vi "Save Report.vi"(8 "error in (no error)":errorcluster, 10 "Results File Location:":path, 11 "NI_report in":refnum<class "NI_report.lvclass">) -> (0 "error out":errorcluster, 1 "generated path":path, 2 "appended path":path, 3 "NI_report out":refnum<class "NI_report.lvclass">)   [LabVIEW 2018]
uses:
  <vilib>/Utility/NIReport.llb/NI_report.lvclass
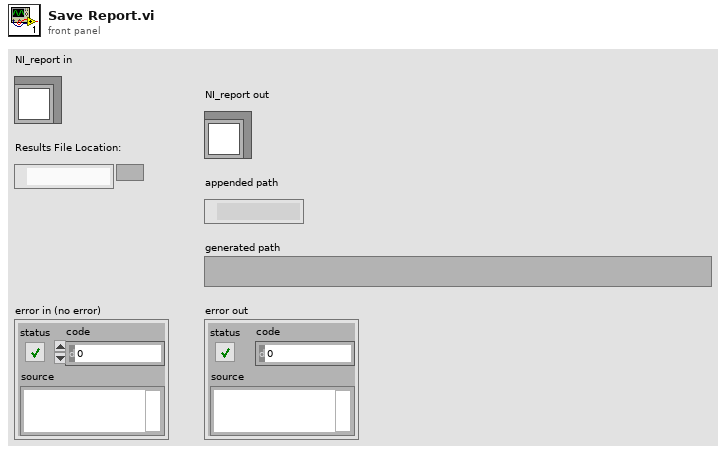
[diagram p1: front panel]
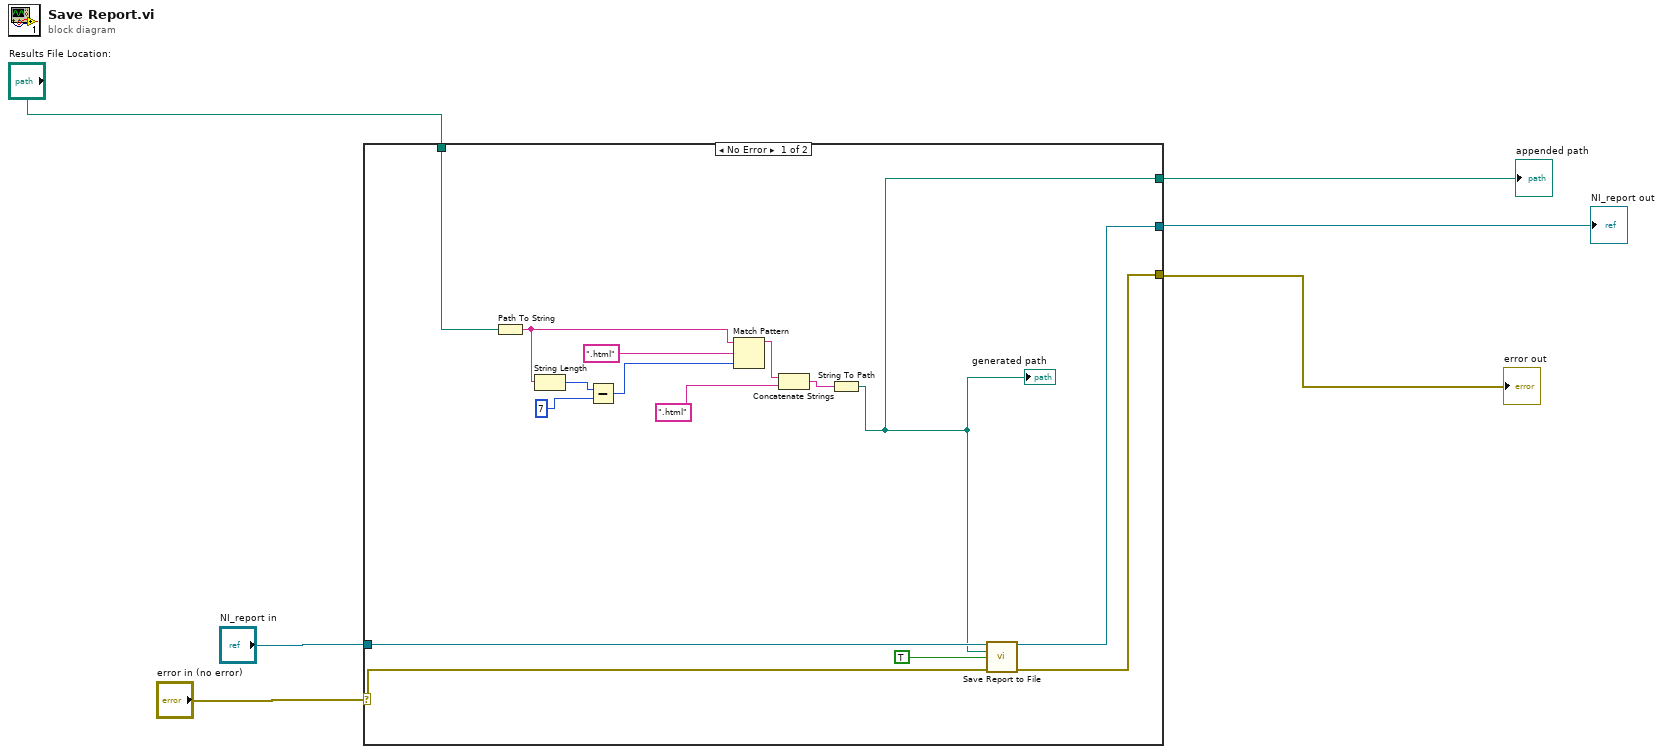
[diagram p0: block diagram]
diagram:
  n1 = case shown="No Error" "error in (no error)" {
    selector: "error in (no error)" -> [w18 w23]
    tunnel: [w19 w23] -> w3
    tunnel: "NI_report in" -> [w21 w22]
    tunnel: [w8 _] -> w1
    tunnel: [w20 w22] -> w4
    tunnel: "Results File Location:" -> [w17 _]
    frame No Error {
      n2 = Path To String(path=w17) -> (string=w13:string)
      n3 = String Length(string=w13) -> (length=w11:i32)
      n4 = Subtract(x=w11, y=7) -> (x-y=w10:i32)
      n5 = Match Pattern(string=w13, regular expression=".html", offset (0)=w10) -> (before substring=w15:string)  [unwired: 3 out]
      n6 = Concatenate Strings(w15, ".html") -> (w9:string)
      n7 = String To Path(string=w9) -> (path=w8:path)
      "generated path" <- w8
      n8 = call-dynamic "Save Report to File.vi"("report in"=w21, "report file path"=w8, "prompt to replace? (F)"=TRUE, "error in (no error)"=w18) -> ("report out"=w20:refnum<class "NI_report.lvclass">, "error out"=w19:errorcluster)  [unwired: 10 in]
    }
    frame Error {
    }
  }
  "NI_report out" <- w4
  "appended path" <- w1
  "error out" <- w3
